vi "黑盾空调.vi"() -> ()   [LabVIEW 2016, in "环境动力监测库.lvlib" / "空调库.lvlib"]
uses:
  <vilib>/ptbypt/NI_PtbyPt.lvlib
panel:
  out "x+1":u32
  out "机柜空调告警状态":T1
  out "开关量输入状态解析":T2
  in  "解除告警":bool
  out "串口":string
  out "传感器状态":T3 {"系统模拟量量化数据"."电流" format="%#.2g"}
  in  "查看型号":bool
  in  "重开串口":bool
  in  "校时":bool
  in  "设定参数":bool
  in  "遥控":bool
  out "获取设备厂家信息":T4
  out "仪器时间":timestamp format="%<%Y/%m/%d %H:%M:%S>T"
  out "系统参数":T5
  out "写入缓冲区":string
  out "读取缓冲区":string
  out "读取选择":string(combo)
  out "通讯":bool=TRUE
  # "℃"
  # "℃"
  # "V"
  # "A"
  # "℃"
  # "℃"
  # "℃"
  # "℃"
  # "℃"
  # "℃"
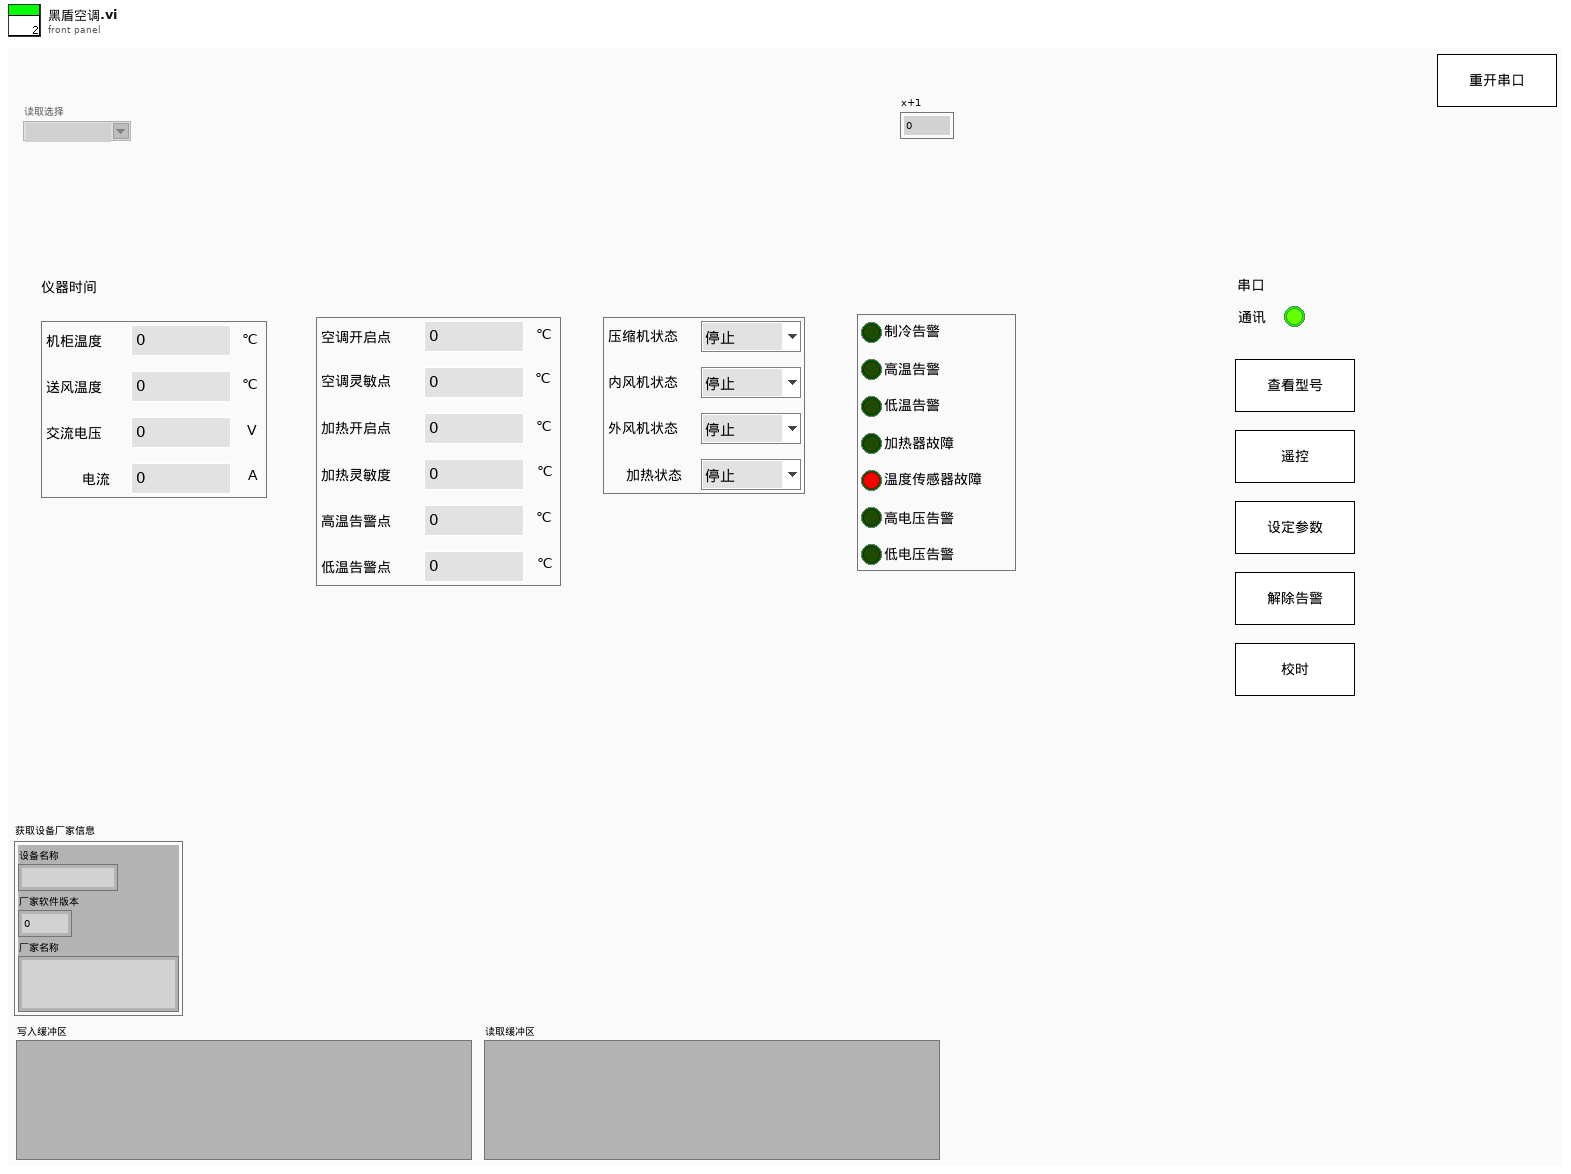
[diagram p1: front panel]
types:
  T1 = cluster{"制冷告警":bool, "高温告警":bool, "低温告警":bool, "加热器故障":bool, "温度传感器故障":bool, "高电压告警":bool, "低电压告警":bool, "预留":u16}
  T2 = cluster{"压缩机状态":enum16{"停止", "运行"}, "内风机状态":enum16{"停止", "运行"}, "外风机状态":enum16{"停止", "运行"}, "加热状态":enum16{"停止", "运行"}}
  T3 = cluster{"系统模拟量量化数据":cluster{"机柜温度":sgl, "送风温度":sgl, "交流电压":sgl, "电流":sgl}}
  T4 = cluster{"设备名称":string, "厂家软件版本":u16, "厂家名称":string}
  T5 = cluster{"空调开启点":u16, "空调灵敏点":u16, "加热开启点":u16, "加热灵敏度":u16, "高温告警点":u16, "低温告警点":u16}
  T6 = cluster{"分支":enum16{"open", "read", "write", "close"}, "字符串":string}
  T7 = cluster{"分支":enum16{"open", "read", "write", "close"}, "读取选择":string}
  T8 = cluster{"型号选择":enum16{"黑盾", "英维克", "仁科测控RS-KTC-N01"}, "MB session in":refnum<class "MB_Master.lvclass">, "英维克空调寄存器":u16[], "通讯状态":bool, "PORT":string, "IP":string, "Slave ID ":u8, "Serial Config":cluster{"baud rate (bps)":u32, "stop bits":u16, "parity":u16, "flow control":u16, "timeout":u32, "retries":i32}, "VISA Resource":refnum<visa-resource-name>, "MB通信方式选择":enum16{"串口", "TCP"}, "系统参数":cluster{"空调开启点":u16, "空调灵敏点":u16, "加热开启点":u16, "加热灵敏度":u16, "高温告警点":u16, "低温告警点":u16}}
  T9 = cluster{"温湿度":cluster{"状态":bool, "温度:":sgl, "湿度:":sgl, "详情  ":bool}, "空调":cluster{"状态":bool, "机柜温度:":sgl, "压缩机:":enum16{"停止", "运行"}, "电加热:":enum16{"停止", "运行"}, "详情  ":bool}, "排气扇":cluster{"排气扇":bool, "详情  ":bool}, "冰箱":cluster{"冰箱":bool, "详情  ":bool}}
  T10 = cluster{"漏水监测输出":cluster{"漏水监测告警":bool, "告警内容":string}, "门禁监测输出":cluster{"门禁监测告警":bool, "告警内容":string}, "门禁监测输出2":cluster{"门禁监测告警":bool, "告警内容":string}, "温湿度监测输出":cluster{"温湿度监测告警":bool, "告警内容":string}, "烟雾监测输出":cluster{"烟雾监测告警":bool, "告警内容":string}, "空调监测输出":cluster{"空调监测告警":bool, "告警内容":string}, "自动重合闸输出":cluster{"自动重合闸告警":bool, "告警内容":string}, "红外入侵输出":cluster{"红外入侵告警":bool, "告警内容":string}, "振动输出":cluster{"振动告警":bool, "告警内容":string}, "UPS输出":cluster{"UPS告警":bool, "告警内容":string}, "蓄电池输出":cluster{"蓄电池告警":bool, "告警内容":string}, "蓄电池输出2":cluster{"蓄电池告警":bool, "告警内容":string}, "GPS输出":cluster{"定位告警":bool, "告警内容":string}, "北斗输出":cluster{"定位告警":bool, "告警内容":string}, "气象输出":cluster{"气象告警":bool, "告警内容":string}, "废液输出":cluster{"废液告警":bool, "告警内容":string}, "废液输出2":cluster{"废液告警":bool, "告警内容":string}}
  T11 = enum32{"Bad", "Idle", "Run top level", "Running"}
  T12 = cluster{"机柜温度":sgl, "送风温度":sgl, "交流电压":sgl, "电流":sgl}
  T13 = cluster{"空调状态":enum16{"停止", "运行"}, "内风机状态":enum16{"停止", "运行"}, "外风机状态":enum16{"停止", "运行"}, "加热状态":enum16{"停止", "运行"}}
  T14 = enum16{"获取模拟量量化数据（浮点数）", "获取模拟量量化数据（定点数）", "获取开关输入状态", "获取机柜空调告警状态", "遥控", "获取系统参数（浮点数）", "获取系统参数（定点数）", "设定系统参数（浮点数）", "设定系统参数（定点数）", "获取系统历史数据（浮点数）", "获取系统历史数据（定点数）", "获取历史告警", "获取监测模块时间", "设定监测模块时间", "获取通信协议版本号", "获取设备地址", "获取设备厂家信息", "设定设备地址（ADR）"}
  T15 = enum16{"空调开机", "空调关机", "制冷开启", "制冷关闭", "制热开启", "制热关闭"}
  T16 = cluster{"分支":enum16{"open", "read", "write", "close"}, "连接的字符串":string}
  T17 = enum16{"空调开启点", "空调灵敏点", "加热开启点", "加热灵敏度", "高温告警点", "低温告警点"}
  T18 = enum16{"空调开启点", "空调灵敏点", "加热开启点", "加热灵敏度", "高温告警点", "低温告警点"}[]
  T19 = typedef "工况数据.ctl" = cluster{"time":string, "data":cluster{"ups":cluster{"ups":cluster{"input_voltage":ext, "input_frequency":ext, "output_voltage":ext, "output_current":ext, "output_frequency":ext, "output_active_power":ext, "output_apparent_power":ext, "load_rate":ext, "cabinet_temperature":ext, "battery_voltage":ext, "remaining_battery_capacity":ext, "power_on_status":string, "power_supply_mode":string, "fault":bool, "battery_low_voltage":bool, "mains_supply_abnormality":bool}, "启用":bool}, "air_conditioner":cluster{"air_conditioner":cluster{"cabinet_temperature":ext, "air_supply_temperature":ext, "voltage":ext, "current":ext, "compressor_status":string, "Internal_fan_status":string, "external_fan_status":string, "heating_state":string, "refrigeration_state":bool, "high_temperature_alarm":bool, "low_temperature_alarm":bool, "heater_fault":bool, "temperature_sensor_fault":bool, "high_voltage_alarm":bool, "low_voltage_alarm":bool, "refrigeration_start_point":ext, "refrigeration_sensitive_point":ext, "heating_start_point":ext, "heating_sensitive_point":ext, "high_temperature_alarm_point":ext, "low_temperature_alarm_point":ext}, "启用":bool}, "smoke_sensor":cluster{"smoke_sensor":cluster{"trigger_alarm":bool}, "启用":bool}, "water_immersion_sensor":cluster{"water_immersion_sensor":cluster{"trigger_alarm":bool}, "启用":bool}, "temperature_and_humidity_sensor":cluster{"temperature_and_humidity_sensor":cluster{"current_temperature":ext, "current_humidity":ext, "room_temperature_alarm":bool, "humidity_alarm":bool}, "启用":bool}, "gps":cluster{"gps":cluster{"current_longitude":ext, "current_latitude":ext, "launch_longitude":ext, "launch_latitude":ext, "shift_alarm":bool}, "启用":bool}, "solar_controller":cluster{"solar_controller":cluster{"array_voltage":ext, "array_current":ext, "generating_power":ext, "battery_voltage":dbl, "battery_current":ext, "ceiling_voltage":ext, "minimum_voltage":ext, "battery_temperature":ext, "remaining_battery_capacity":ext, "load_voltage":ext, "load_current":ext, "load_power":ext, "equipment_temperature":ext, "accumulated_electricity_consumption_of_the_day":ext, "accumulated_electricity_consumption_of_the_current_month":ext, "accumulated_electricity_consumption_in_the_current_year":ext, "total_accumulated_power_consumption":ext, "accumulated_charging_capacity_of_the_day":ext, "accumulated_charging_amount_of_the_current_month":ext, "accumulated_charging_capacity_of_the_current_year":ext, "total_cumulative_charge":ext}, "启用":bool}, "solar_controller_2":cluster{"solar_controller_2":cluster{"array_voltage":ext, "array_current":ext, "generating_power":ext, "battery_voltage":dbl, "battery_current":ext, "ceiling_voltage":ext, "minimum_voltage":ext, "battery_temperature":ext, "remaining_battery_capacity":ext, "load_voltage":ext, "load_current":ext, "load_power":ext, "equipment_temperature":ext, "accumulated_electricity_consumption_of_the_day":ext, "accumulated_electricity_consumption_of_the_current_month":ext, "accumulated_electricity_consumption_in_the_current_year":ext, "total_accumulated_power_consumption":ext, "accumulated_charging_capacity_of_the_day":ext, "accumulated_charging_amount_of_the_current_month":ext, "accumulated_charging_capacity_of_the_current_year":ext, "total_cumulative_charge":ext}, "启用":bool}, "NH3":cluster{"NH3":cluster{"F0":ext, "F1":ext, "syringe_temperature":ext, "alarm_step":dbl, "X0":ext}, "启用":bool}, "TP":cluster{"TP":cluster{"F0":ext, "F1":ext, "F2":ext, "F3":ext, "digestion_temperature":ext, "constant_temperature":ext, "syringe_temperature":ext, "alarm_step":dbl, "X0":ext}, "启用":bool}, "TN":cluster{"TN":cluster{"F0":ext, "F1":ext, "F2":ext, "F3":ext, "F4":ext, "F5":ext, "F6":ext, "F7":ext, "digestion_temperature":ext, "constant_temperature":ext, "syringe_temperature":ext, "alarm_step":dbl, "X0":ext}, "启用":bool}, "CODMn":cluster{"CODMn":cluster{"temperature_curve":ext[], "titration_curve":ext[], "F0":ext, "F1":ext, "F2":ext, "F3":ext, "F4":ext, "F5":ext, "A":ext, "B":ext, "K":ext}, "启用":bool}, "CODCr":cluster{"CODCr":cluster{"temperature_curve":ext[], "F0":ext, "F1":ext, "reagent_sensor":ext}, "启用":bool}}}
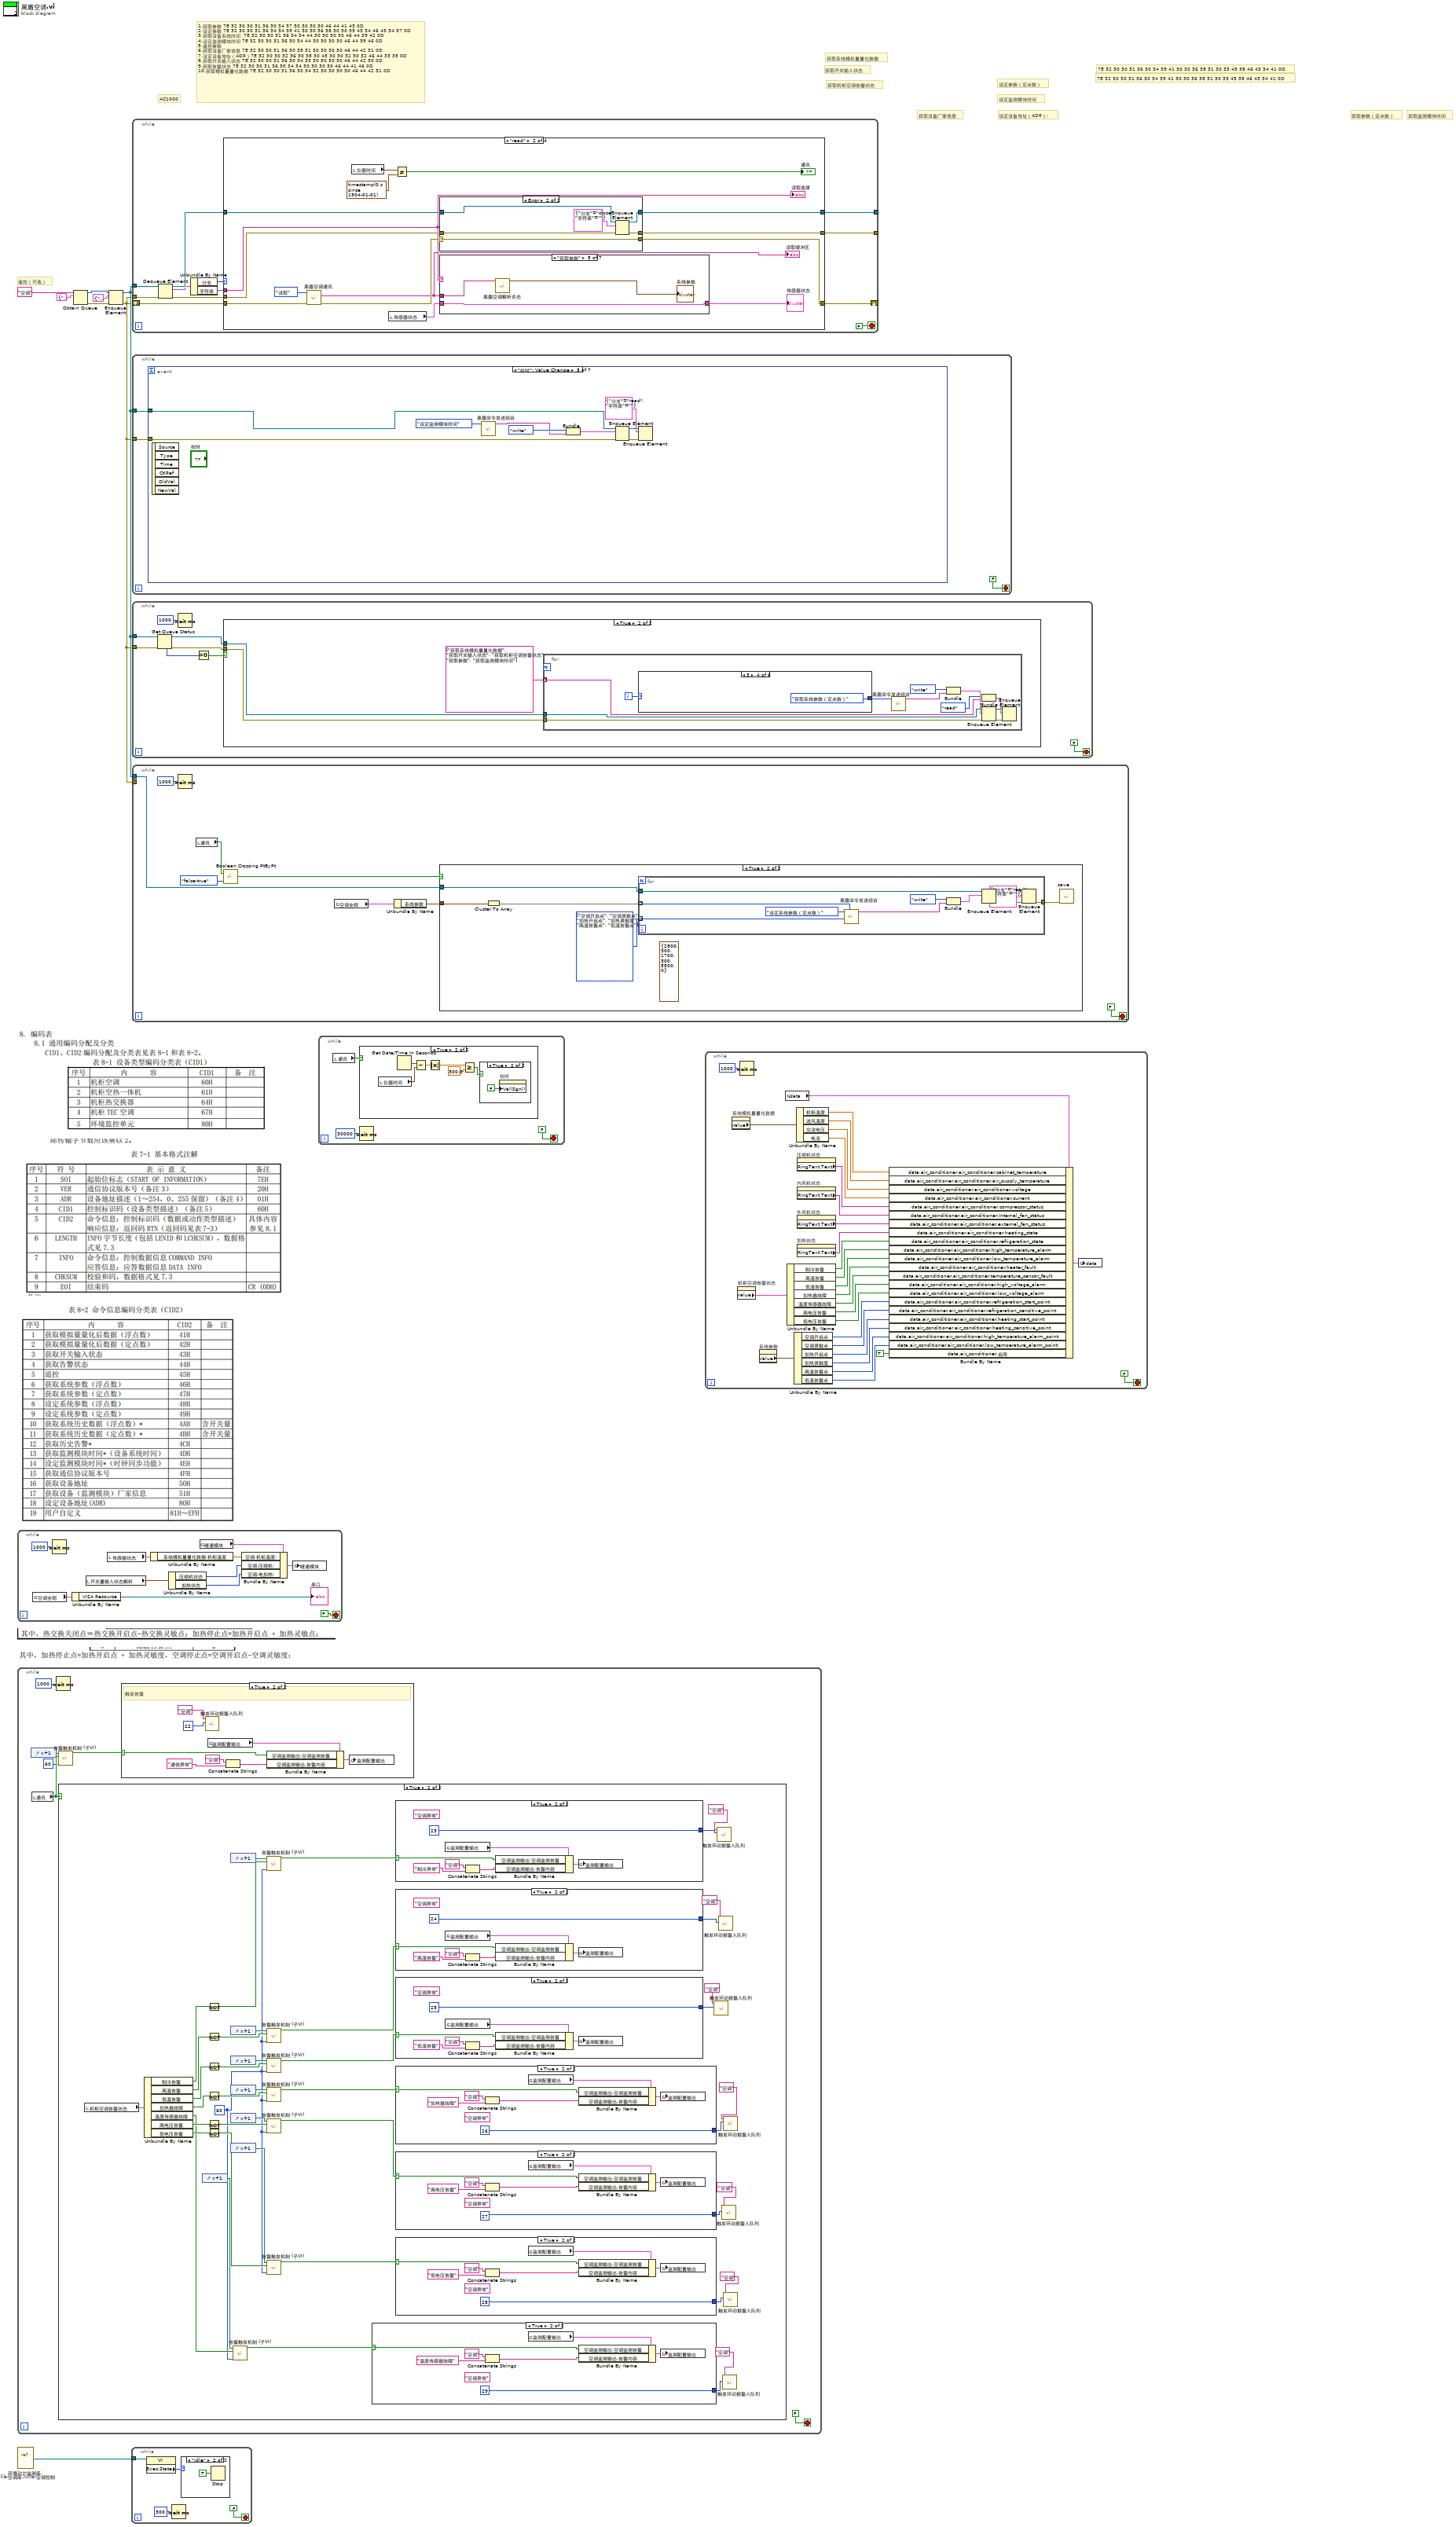
[diagram p0: block diagram]
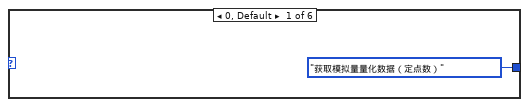
[diagram p16: hidden frame]
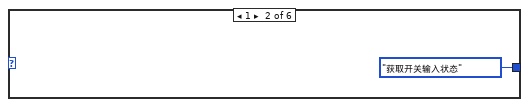
[diagram p17: hidden frame]
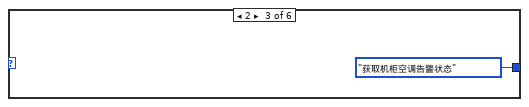
[diagram p18: hidden frame]
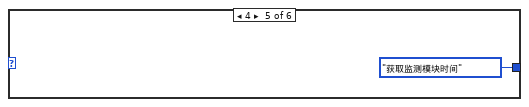
[diagram p19: hidden frame]
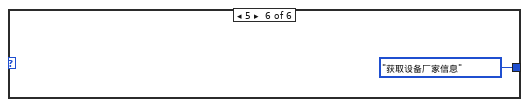
[diagram p20: hidden frame]
diagram:
  # "获取系统模拟量量化数据"
  # "设定设备地址（ADR）:"
  # "获取设备厂家信息"
  # "设定监测模块时间"
  # "获取监测模块时间"
  # "设定参数（定点数）"
  # "获取参数（定点数）"
  # "遥控（可选）"
  # "获取机柜空调告警状态"
  # "获取开关输入状态"
  # "7E 32 30 30 31 36 30 34 39 41 30 30 36 38 31 30 33 45 38 46 43 34 41 0D"
  # "7E 32 30 30 31 36 30 34 39 41 30 30 36 38 31 30 33 45 38 46 43 34 41 0D"
  # "AC1000"
  # "1.获取参数 7E 32 30 30 31 36 30 34 37 30 30 30 30 46 44 41 43 0D\n2.设定参数 7E 32 30 30 31 36 34 34 39 41 30 30 36 38 30 30 39 43 34 46 43 34 37 0D \n3.获取设备系统时间  7E 32 30 30 31 36 34 34 44 30 30 30 30 46 44 39 42 0D\n4.设定监测模块时间 7E 32 30 30 31 36 30 34 44 30 30 30 30 46 44 39 46 0D\n5.遥控参数\n6.获取设备厂家信息 7E 32 30 30 31 36 30 35 31 30 30 30 30 46 44 42 31 0D\n7.设定设备地址（ADR）7E 32 30 30 32 36 30 38 30 45 30 30 32 30 32 46 44 33 35 0D\n8.获取开关输入状态 7E 32 30 30 31 36 30 34 33 30 30 30 30 46 44 42 30 0D\n9.获取告警状态 7E 32 30 30 31 36 30 34 34 30 30 30 30 46 44 41 46 0D\n10.获取模拟量量化数据 7E 32 30 30 31 36 30 34 32 30 30 30 30 46 44 42 31 0D"
  n1 = while {
    stop <- FALSE stop-if-true
    n2 = global read "断电保存全局变量.vi" "空调全局"() -> (w10:T8)
    n3 = Wait (ms)(milliseconds to wait=u32 1000 ("等待时间（毫秒）")) -> ()  [unwired: 1 out]
    n4 = Unbundle By Name(w10) -> ("VISA Resource"=→"串口":refnum<visa-resource-name>)
    n5 = local read "开关量输入状态解析"() -> (w15:T2)
    n6 = local read "传感器状态"() -> (w13:T3)
    n7 = Unbundle By Name(w13) -> ("系统模拟量量化数据.机柜温度"=w14:sgl)
    n8 = Unbundle By Name(w15) -> ("压缩机状态"=w16:enum16{"停止", "运行"}, "加热状态"=w17:enum16{"停止", "运行"})
    n9 = global read "内部交互全局变量.vi" "暖通模块"() -> (w11:T9)
    n10 = Bundle By Name(cluster=w11, "空调.机柜温度:"=w14, "空调.压缩机:"=w16, "空调.电加热:"=w17) -> (w12:T9)
    n11 = global write "内部交互全局变量.vi" "暖通模块"(w12) -> ()
  }
  n12 = while {
    stop <- FALSE stop-if-true
    n13 = control-ref of="x+1"() -> (w21:refnum<vi>)
    n14 = local read "通讯"() -> (w22:bool)
    n15 = Wait (ms)(milliseconds to wait=u32 1000 ("等待时间（毫秒）")) -> ()  [unwired: 1 out]
    n16 = call "告警触发机制 (子VI).vi"("信号持续时间"=u32 60, "状态输出真-正常"=w22, "Digital输入"=w21) -> ("触发告警"=w23:bool)  [unwired: 6 in, 2 out]
    n17 = case shown="True" w22 {
      frame False {
      }
      frame True {
        w40 = u32 60 ("信号持续时间")
        n18 = local read "机柜空调告警状态"() -> (w68:T1)
        n19 = Unbundle By Name(w68) -> ("制冷告警"=w64:bool, "高温告警"=w58:bool, "低温告警"=w55:bool, "加热器故障"=w51:bool, "温度传感器故障"=w42:bool, "高电压告警"=w47:bool, "低电压告警"=w45:bool)
        n20 = control-ref of="x+1"() -> (w43:refnum<vi>)
        n21 = Not(x=w64) -> (.not. x?=w65:bool)
        n22 = Not(x=w58) -> (.not. x?=w61:bool)
        n23 = Not(x=w55) -> (.not. x?=w57:bool)
        n24 = Not(x=w51) -> (.not. x?=w53:bool)
        n25 = Not(x=w47) -> (.not. x?=w49:bool)
        n26 = Not(x=w45) -> (.not. x?=w62:bool)
        n27 = control-ref of="x+1"() -> (w66:refnum<vi>)
        n28 = control-ref of="x+1"() -> (w60:refnum<vi>)
        n29 = control-ref of="x+1"() -> (w56:refnum<vi>)
        n30 = control-ref of="x+1"() -> (w52:refnum<vi>)
        n31 = control-ref of="x+1"() -> (w48:refnum<vi>)
        n32 = control-ref of="x+1"() -> (w67:refnum<vi>)
        n33 = call "告警触发机制 (子VI).vi"("信号持续时间"=w40, "状态输出真-正常"=w42, "Digital输入"=w43) -> ("触发告警"=w41:bool)  [unwired: 6 in, 2 out]
        n34 = call "告警触发机制 (子VI).vi"("信号持续时间"=w40, "状态输出真-正常"=w65, "Digital输入"=w66) -> ("触发告警"=w63:bool)  [unwired: 6 in, 2 out]
        n35 = call "告警触发机制 (子VI).vi"("信号持续时间"=w40, "状态输出真-正常"=w61, "Digital输入"=w60) -> ("触发告警"=w59:bool)  [unwired: 6 in, 2 out]
        n36 = call "告警触发机制 (子VI).vi"("信号持续时间"=w40, "状态输出真-正常"=w57, "Digital输入"=w56) -> ("触发告警"=w54:bool)  [unwired: 6 in, 2 out]
        n37 = call "告警触发机制 (子VI).vi"("信号持续时间"=w40, "状态输出真-正常"=w53, "Digital输入"=w52) -> ("触发告警"=w50:bool)  [unwired: 6 in, 2 out]
        n38 = call "告警触发机制 (子VI).vi"("信号持续时间"=w40, "状态输出真-正常"=w49, "Digital输入"=w48) -> ("触发告警"=w46:bool)  [unwired: 6 in, 2 out]
        n39 = call "告警触发机制 (子VI).vi"("信号持续时间"=w40, "状态输出真-正常"=w62, "Digital输入"=w67) -> ("触发告警"=w44:bool)  [unwired: 6 in, 2 out]
        n40 = case shown="True" w41 {
          selector: w41 -> [_ w86]
          tunnel: [_ 29 ("code")] -> w26
          frame False {
          }
          frame True {
            (unwired) "空调异常" ("设备")
            n41 = Concatenate Strings("空调" ("设备"), "温度传感器故障" ("日志信息")) -> (w85:string)
            n42 = global read "内部交互全局变量.vi" "监测配置输出"() -> (w88:T10)
            n43 = Bundle By Name(cluster=w88, "空调监测输出.空调监测告警"=w86, "空调监测输出.告警内容"=w85) -> (w87:T10)
            n44 = global write "内部交互全局变量.vi" "监测配置输出"(w87) -> ()
          }
        }
        n45 = case shown="True" w63 {
          selector: w63 -> [_ w114]
          tunnel: [_ 23 ("code")] -> w39
          frame False {
          }
          frame True {
            (unwired) "空调异常" ("设备")
            n46 = global read "内部交互全局变量.vi" "监测配置输出"() -> (w116:T10)
            n47 = Concatenate Strings("空调" ("设备"), "制冷异常" ("日志信息")) -> (w113:string)
            n48 = Bundle By Name(cluster=w116, "空调监测输出.空调监测告警"=w114, "空调监测输出.告警内容"=w113) -> (w115:T10)
            n49 = global write "内部交互全局变量.vi" "监测配置输出"(w115) -> ()
          }
        }
        n50 = case shown="True" w59 {
          selector: w59 -> [_ w107]
          tunnel: [_ 24 ("code")] -> w36
          frame False {
          }
          frame True {
            (unwired) "空调异常" ("设备")
            n51 = global read "内部交互全局变量.vi" "监测配置输出"() -> (w109:T10)
            n52 = Concatenate Strings("空调" ("设备"), "高温告警" ("日志信息")) -> (w106:string)
            n53 = Bundle By Name(cluster=w109, "空调监测输出.空调监测告警"=w107, "空调监测输出.告警内容"=w106) -> (w108:T10)
            n54 = global write "内部交互全局变量.vi" "监测配置输出"(w108) -> ()
          }
        }
        n55 = case shown="True" w54 {
          selector: w54 -> [_ w100]
          tunnel: [_ 25 ("code")] -> w35
          frame False {
          }
          frame True {
            (unwired) "空调异常" ("设备")
            n56 = global read "内部交互全局变量.vi" "监测配置输出"() -> (w102:T10)
            n57 = Concatenate Strings("空调" ("设备"), "低温告警" ("日志信息")) -> (w99:string)
            n58 = Bundle By Name(cluster=w102, "空调监测输出.空调监测告警"=w100, "空调监测输出.告警内容"=w99) -> (w101:T10)
            n59 = global write "内部交互全局变量.vi" "监测配置输出"(w101) -> ()
          }
        }
        n60 = case shown="True" w50 {
          selector: w50 -> [_ w93]
          tunnel: [_ 26 ("code")] -> w32
          frame False {
          }
          frame True {
            (unwired) "空调异常" ("设备")
            n61 = Concatenate Strings("空调" ("设备"), "加热器故障" ("日志信息")) -> (w92:string)
            n62 = global read "内部交互全局变量.vi" "监测配置输出"() -> (w95:T10)
            n63 = Bundle By Name(cluster=w95, "空调监测输出.空调监测告警"=w93, "空调监测输出.告警内容"=w92) -> (w94:T10)
            n64 = global write "内部交互全局变量.vi" "监测配置输出"(w94) -> ()
          }
        }
        n65 = case shown="True" w46 {
          selector: w46 -> [_ w79]
          tunnel: [_ 27 ("code")] -> w31
          frame False {
          }
          frame True {
            (unwired) "空调异常" ("设备")
            n66 = Concatenate Strings("空调" ("设备"), "高电压告警" ("日志信息")) -> (w78:string)
            n67 = global read "内部交互全局变量.vi" "监测配置输出"() -> (w81:T10)
            n68 = Bundle By Name(cluster=w81, "空调监测输出.空调监测告警"=w79, "空调监测输出.告警内容"=w78) -> (w80:T10)
            n69 = global write "内部交互全局变量.vi" "监测配置输出"(w80) -> ()
          }
        }
        n70 = case shown="True" w44 {
          selector: w44 -> [_ w71]
          tunnel: [_ 28 ("code")] -> w28
          frame False {
          }
          frame True {
            (unwired) "空调异常" ("设备")
            n71 = Concatenate Strings("空调" ("设备"), "低电压告警" ("日志信息")) -> (w72:string)
            n72 = global read "内部交互全局变量.vi" "监测配置输出"() -> (w74:T10)
            n73 = Bundle By Name(cluster=w74, "空调监测输出.空调监测告警"=w71, "空调监测输出.告警内容"=w72) -> (w73:T10)
            n74 = global write "内部交互全局变量.vi" "监测配置输出"(w73) -> ()
          }
        }
        n75 = call "触发环动报警入队列.vi"("code"=w35, "元器件"="空调") -> ()  [unwired: 10 in]
        n76 = call "触发环动报警入队列.vi"("code"=w39, "元器件"="空调") -> ()  [unwired: 10 in]
        n77 = call "触发环动报警入队列.vi"("code"=w36, "元器件"="空调") -> ()  [unwired: 10 in]
        n78 = call "触发环动报警入队列.vi"("code"=w31, "元器件"="空调") -> ()  [unwired: 10 in]
        n79 = call "触发环动报警入队列.vi"("code"=w26, "元器件"="空调") -> ()  [unwired: 10 in]
        n80 = call "触发环动报警入队列.vi"("code"=w32, "元器件"="空调") -> ()  [unwired: 10 in]
        n81 = call "触发环动报警入队列.vi"("code"=w28, "元器件"="空调") -> ()  [unwired: 10 in]
      }
    }
    n82 = case shown="True" w23 {
      selector: w23 -> [_ w125]
      frame False {
      }
      frame True {
        # "触发告警"
        n83 = call "触发环动报警入队列.vi"("code"=22, "元器件"="空调" ("设备")) -> ()  [unwired: 10 in]
        n84 = global read "内部交互全局变量.vi" "监测配置输出"() -> (w124:T10)
        n85 = Concatenate Strings("空调" ("设备"), "通信异常" ("设备")) -> (w121:string)
        n86 = Bundle By Name(cluster=w124, "空调监测输出.空调监测告警"=w125, "空调监测输出.告警内容"=w121) -> (w123:T10)
        n87 = global write "内部交互全局变量.vi" "监测配置输出"(w123) -> ()
      }
    }
  }
  n88 = vi-ref "环境动力监测库.lvlib:空调库.lvlib:空调控制.vi"() -> (w3:refnum<vi>)
  n89 = Obtain Queue(name (unnamed)="空调" ("名称（未命名）"), element data type=T6 {"分支"=enum."open", "字符串"="获取系统模拟量量化数据"}) -> (queue out=w7:refnum<queue>, error out=w6:errorcluster)  [unwired: 3 in, 1 out]
  n90 = Enqueue Element(queue=w7, element=T7 {"分支"=enum."open", "读取选择"="获取系统模拟量量化数据"}, error in (no error)=w6) -> (queue out=w2:refnum<queue>, error out=w1:errorcluster)  [unwired: 1 in, 1 out]
  n91 = while {
    tunnel: w3 -> [w129]
    stop <- FALSE stop-if-true
    n92 = property class="VI"(reference=w129) -> ("Exec.State"=w128:T11)  [unwired: 1 in, 2 out]
    n93 = Wait (ms)(milliseconds to wait=u32 300 ("等待时间（毫秒）")) -> ()  [unwired: 1 out]
    n94 = case shown="\"Idle\"" w128 {
      frame "Bad", Default {
      }
      frame "Idle" {
        n95 = Stop(stop? (T)=TRUE ("停止？(T)")) -> ()
      }
    }
  }
  n96 = while {
    tunnel: w2 -> [w141]
    tunnel: w1 -> [w140]
    shift-right: [w139] -> _
    shift-left: w1 -> [w138]
    tunnel: [w135] -> _
    tunnel: [w134] -> _
    stop <- FALSE stop-if-true
    n97 = Dequeue Element(queue=w141, error in (no error)=w140) -> (queue out=w137:refnum<queue>, element=w133:T6, error out=w136:errorcluster)  [unwired: 1 in, 1 out]
    n98 = Unbundle By Name(w133) -> ("分支"=w132:enum16{"open", "read", "write", "close"}, "字符串"=w131:string)
    n99 = case shown="\"read\"" w132 {
      tunnel: [w147 w154 w196 w204] -> w139
      tunnel: w138 -> [_ w162 w197 w205]
      tunnel: w137 -> [w146 w158 w194 w203]
      tunnel: w136 -> [w145 w156 w193 w202]
      tunnel: [w146 w157 w194 w200] -> w135
      tunnel: [w145 w155 w193 w199] -> w134
      tunnel: w131 -> [_ w161 w195 _]
      frame "open", Default {
        n100 = global read "断电保存全局变量.vi" "空调全局"() -> (w144:T8)
        n101 = Unbundle By Name(w144) -> ("VISA Resource"=w143:refnum<visa-resource-name>)
        n102 = call "黑盾空调通讯.vi"("VISA resource name"=w143, "功能输入"=enum16{"打开串口", "写入", "读取", "关闭串口"}."打开串口") -> ("error out"=w147:errorcluster)  [unwired: 7 in, 2 out]
      }
      frame "read" {
        n103 = call "黑盾空调通讯.vi"("error in (no error)"=w162, "功能输入"=enum16{"打开串口", "写入", "读取", "关闭串口"}."读取") -> ("error out"=w159:errorcluster, "读取缓冲区"=w153:string)  [unwired: 7 in, 1 out]
        "读取缓冲区" <- w153
        n104 = local read "仪器时间"() -> (w149:timestamp)
        n105 = local read "传感器状态"() -> (w160:T3)
        n106 = Not Equal?(x=w149, y=timestamp(0 s since 1904-01-01)) -> (x != y?=→"通讯":bool)
        n107 = case shown="Error" w159 {
          selector: w159 -> [w166 w167]
          tunnel: w158 -> [w165 w171]
          tunnel: [w165 w170] -> w157
          tunnel: w156 -> [w164 w169]
          tunnel: [w164 w168] -> w155
          tunnel: [w166 w167] -> w154
          frame No Error {
          }
          frame Error {
            n108 = Enqueue Element(queue=w171, element=T6 {"分支"=enum."close", "字符串"=""} ("元素"), error in (no error)=w169) -> (queue out=w170:refnum<queue>, error out=w168:errorcluster)  [unwired: 1 in, 1 out]
          }
        }
        n109 = case shown="\"获取参数\"" w161 {
          tunnel: w153 -> [_ w177 w180 w183 w186 w189 w192]
          tunnel: w160 -> [w173 w176 w178 w182 w184 w188 w190]
          tunnel: [w173 w174 w178 w182 w184 w188 w190] -> w152
          frame "假", Default {
          }
          frame "获取系统模拟量量化数据" {
            n110 = call-poly "黑盾空调解析多态.vi"("输入字符串"=w177) -> ("系统模拟量量化数据"=w175:T12)  [unwired: 10 in]
            n111 = Bundle By Name(cluster=w176, "系统模拟量量化数据"=w175) -> (w174:T3)
          }
          frame "获取开关输入状态" {
            n112 = call-poly "黑盾空调解析多态.vi"("输入字符串"=w180) -> ("开关量输入状态解析"=→"开关量输入状态解析":T13)  [unwired: 10 in]
          }
          frame "获取机柜空调告警状态" {
            n113 = call-poly "黑盾空调解析多态.vi"("输入字符串"=w183) -> ("机柜空调告警状态"=→"机柜空调告警状态":T1)  [unwired: 10 in]
          }
          frame "获取参数" {
            n114 = call-poly "黑盾空调解析多态.vi"("输入字符串"=w186) -> ("获取参数(定点数)"=→"系统参数":T5)  [unwired: 10 in]
          }
          frame "获取监测模块时间" {
            n115 = call-poly "黑盾空调解析多态.vi"("输入字符串"=w189) -> ("时间标识"=→"仪器时间":timestamp)  [unwired: 10 in]
          }
          frame "获取设备厂家信息" {
            n116 = call-poly "黑盾空调解析多态.vi"("输入字符串"=w192) -> ("获取设备厂家信息"=→"获取设备厂家信息":T4)  [unwired: 10 in]
          }
        }
        "传感器状态" <- w152
        "读取选择" <- w161
      }
      frame "write" {
        n117 = call "黑盾空调通讯.vi"("error in (no error)"=w197, "写入缓冲区"=w195, "功能输入"=enum16{"打开串口", "写入", "读取", "关闭串口"}."写入") -> ("error out"=w196:errorcluster)  [unwired: 6 in, 2 out]
        "写入缓冲区" <- w195
      }
      frame "close" {
        n118 = call "黑盾空调通讯.vi"("error in (no error)"=w205, "功能输入"=enum16{"打开串口", "写入", "读取", "关闭串口"}."关闭串口") -> ("error out"=w204:errorcluster)  [unwired: 7 in, 2 out]
        n119 = Enqueue Element(queue=w203, element=T6 {"分支"=enum."open", "字符串"=""} ("元素"), error in (no error)=w202) -> (queue out=w200:refnum<queue>, error out=w199:errorcluster)  [unwired: 1 in, 1 out]
      }
    }
  }
  n120 = while {
    tunnel: w2 -> [w208]
    tunnel: w1 -> [w207]
    stop <- FALSE stop-if-true
    n121 = event shown="[4] \"校时\": Value Change" {
      selector: _ -> [_ _ _ _ _ _ _]
      dyn-events: _ -> [_ _ _ _ _ _ _]
      timeout: _ -> [_ _ _ _ _ _ _]
      tunnel: w208 -> [_ w215 w234 w253 w288 _ _]
      tunnel: w207 -> [_ w214 w235 w252 w287 _ _]
      event Timeout {
        n122 = event-data() -> ()  [unwired: 1 in, 3 out]
      }
      event "重开串口": Value Change {
        n123 = event-data() -> ()  [unwired: 1 in, 6 out]
        n124 = global read "断电保存全局变量.vi" "空调全局"() -> (w210:T8)
        n125 = Unbundle By Name(w210) -> ("VISA Resource"=w213:refnum<visa-resource-name>, "IP"=w212:string, "PORT"=w211:string)
        n126 = call "串口配置.vi"("PORT"=w211, "IP"=w212, "请选择串口:"=w213) -> ("PORT 2"=w216:string, "IP 2"=w217:string, "确认 2"=w218:bool, "VISA资源名称 2"=w219:refnum<visa-resource-name>)  [unwired: 5 in]
        n127 = case shown="True" w218 {
          tunnel: w219 -> [_ w223]
          tunnel: w215 -> [_ w225]
          tunnel: w214 -> [_ w224]
          tunnel: w217 -> [_ w222]
          tunnel: w216 -> [_ w221]
          tunnel: w210 -> [_ w220]
          frame False {
          }
          frame True {
            n128 = flat-sequence {
              tunnel: w225 -> [w233]
              tunnel: w224 -> [w232]
              tunnel: w223 -> [w229]
              tunnel: w222 -> [w228]
              tunnel: w221 -> [w227]
              tunnel: w220 -> [w230]
              frame #0 {
                n129 = Bundle By Name(cluster=w230, "VISA Resource"=w229, "IP"=w228, "PORT"=w227) -> (w226:T8)
                n130 = global write "断电保存全局变量.vi" "空调全局"(w226) -> ()
                n131 = Enqueue Element(queue=w233, element=T6 {"分支"=enum."close", "字符串"=""} ("元素"), error in (no error)=w232) -> ()  [unwired: 1 in, 3 out]
              }
              frame #1 {
                n132 = call "save.vi"() -> ()  [unwired: 11 in, 1 out]
              }
            }
          }
        }
      }
      event "遥控": Value Change {
        n133 = event-data() -> ()  [unwired: 1 in, 6 out]
        n134 = call "遥控参数对话框.vi"() -> ("遥控参数选择输出"=w236:T15, "确定?"=w237:bool)  [unwired: 10 in]
        n135 = case shown="True" w237 {
          tunnel: w236 -> [_ w246]
          tunnel: w235 -> [_ w245]
          tunnel: w234 -> [_ w244]
          frame False {
          }
          frame True {
            n136 = call "黑盾命令发送组合.vi"("遥控参数选择"=w246, "CID2枚举"=T14."遥控") -> ("连接的字符串"=w242:string)  [unwired: 9 in]
            n137 = Bundle("分支"=enum16{"open", "read", "write", "close"}."write", "连接的字符串"=w242) -> (w241:T16)  [unwired: 1 in]
            n138 = Enqueue Element(queue=w244, element=w241, error in (no error)=w245) -> (queue out=w240:refnum<queue>, error out=w239:errorcluster)  [unwired: 1 in, 1 out]
            n139 = Enqueue Element(queue=w240, element=T6 {"分支"=enum."read", "字符串"=""} ("元素"), error in (no error)=w239) -> ()  [unwired: 1 in, 3 out]
          }
        }
      }
      event "设定参数": Value Change {
        n140 = event-data() -> ()  [unwired: 1 in, 6 out]
        n141 = local read "系统参数"() -> (w248:T5)
        n142 = call "设定参数对话框.vi"("获取参数(定点数)"=w248) -> ("参数 2"=w249:u16, "设定参数（定点数）选择 2"=w250:T17, "确定?"=w251:bool)  [unwired: 8 in]
        n143 = case shown="True" w251 {
          tunnel: w252 -> [_ w263]
          tunnel: w253 -> [_ w262]
          tunnel: w250 -> [_ w255]
          tunnel: w249 -> [_ w254]
          frame False {
          }
          frame True {
            n144 = flat-sequence {
              tunnel: w255 -> [w268]
              tunnel: w254 -> [w265]
              frame #0 {
                n145 = global read "断电保存全局变量.vi" "空调全局"() -> (w267:T8)
                n146 = case shown="\"低温告警点\"" w268 {
                  tunnel: w267 -> [w271 w273 w276 w279 w282 w285]
                  tunnel: w265 -> [w270 w274 w277 w280 w283 w286]
                  tunnel: [w269 w272 w275 w278 w281 w284] -> w266
                  frame "空调开启点", Default {
                    n147 = Bundle By Name(cluster=w271, "系统参数.空调开启点"=w270) -> (w269:T8)
                  }
                  frame "空调灵敏点" {
                    n148 = Bundle By Name(cluster=w273, "系统参数.空调灵敏点"=w274) -> (w272:T8)
                  }
                  frame "加热开启点" {
                    n149 = Bundle By Name(cluster=w276, "系统参数.加热开启点"=w277) -> (w275:T8)
                  }
                  frame "加热灵敏度" {
                    n150 = Bundle By Name(cluster=w279, "系统参数.加热灵敏度"=w280) -> (w278:T8)
                  }
                  frame "高温告警点" {
                    n151 = Bundle By Name(cluster=w282, "系统参数.高温告警点"=w283) -> (w281:T8)
                  }
                  frame "低温告警点" {
                    n152 = Bundle By Name(cluster=w285, "系统参数.低温告警点"=w286) -> (w284:T8)
                  }
                }
                n153 = global write "断电保存全局变量.vi" "空调全局"(w266) -> ()
              }
              frame #1 {
                n154 = call "save.vi"() -> ()  [unwired: 11 in, 1 out]
              }
            }
            n155 = call "黑盾命令发送组合.vi"("参数"=w254, "设定参数（定点数）选择"=w255, "CID2枚举"=T14."设定系统参数（定点数）") -> ("连接的字符串"=w260:string)  [unwired: 8 in]
            n156 = Bundle("分支"=enum16{"open", "read", "write", "close"}."write", "连接的字符串"=w260) -> (w259:T16)  [unwired: 1 in]
            n157 = Enqueue Element(queue=w262, element=w259, error in (no error)=w263) -> (queue out=w258:refnum<queue>, error out=w257:errorcluster)  [unwired: 1 in, 1 out]
            n158 = Enqueue Element(queue=w258, element=T6 {"分支"=enum."read", "字符串"=""} ("元素"), error in (no error)=w257) -> ()  [unwired: 1 in, 3 out]
          }
        }
      }
      event "校时": Value Change {
        n159 = event-data() -> ()  [unwired: 1 in, 6 out]
        n160 = call "黑盾命令发送组合.vi"("CID2枚举"=T14."设定监测模块时间") -> ("连接的字符串"=w293:string)  [unwired: 10 in]
        n161 = Bundle("分支"=enum16{"open", "read", "write", "close"}."write", "连接的字符串"=w293) -> (w292:T16)  [unwired: 1 in]
        n162 = Enqueue Element(queue=w288, element=w292, error in (no error)=w287) -> (queue out=w291:refnum<queue>, error out=w290:errorcluster)  [unwired: 1 in, 1 out]
        n163 = Enqueue Element(queue=w291, element=T6 {"分支"=enum."read", "字符串"=""} ("元素"), error in (no error)=w290) -> ()  [unwired: 1 in, 3 out]
      }
      event "查看型号": Value Change {
        n164 = event-data() -> ()  [unwired: 1 in, 6 out]
        n165 = One Button Dialog(message="空调品牌为:黑盾" ("消息")) -> ()  [unwired: 1 in, 1 out]
      }
      event "解除告警": Value Change {
        n166 = event-data() -> ()  [unwired: 1 in, 6 out]
        n167 = global read "内部交互全局变量.vi" "监测配置输出"() -> (w298:T10)
        n168 = Bundle By Name(cluster=w298, "空调监测输出.空调监测告警"=FALSE) -> (w297:T10)
        n169 = global write "内部交互全局变量.vi" "监测配置输出"(w297) -> ()
        "x+1" <- u32 0 ("x+1")
      }
    }
  }
  n170 = while {
    tunnel: w2 -> [w307]
    tunnel: w1 -> [w306]
    stop <- FALSE stop-if-true
    n171 = Get Queue Status(queue=w307, error in (no error)=w306) -> (queue out=w303:refnum<queue>, error out=w302:errorcluster, # elements in queue=w305:i32)  [unwired: 1 in, 5 out]
    n172 = Wait (ms)(milliseconds to wait=u32 1000 ("等待时间（毫秒）")) -> ()  [unwired: 1 out]
    n173 = Equal To 0?(x=w305) -> (x = 0?=w304:bool)
    n174 = case shown="True" w304 {
      tunnel: w303 -> [_ w310]
      tunnel: w302 -> [_ w309]
      frame False {
      }
      frame True {
        n175 = for {
          tunnel: string[] ["获取系统模拟量量化数据", "获取开关输入状态", "获取机柜空调告警状态", "获取参数", "获取监测模块时间"] -> [w313] mode=indexing
          tunnel: w310 -> [w323]
          tunnel: w309 -> [w322]
          i -> [w321]
          n176 = case shown="3" w321 {
            tunnel: [T14."获取模拟量量化数据（定点数）" ("CID2枚举") T14."获取开关输入状态" ("CID2枚举") T14."获取机柜空调告警状态" ("CID2枚举") T14."获取系统参数（定点数）" ("CID2枚举") T14."获取监测模块时间" ("CID2枚举") T14."获取设备厂家信息" ("CID2枚举")] -> w320
            frame 0, Default {
            }
            frame 1 {
            }
            frame 2 {
            }
            frame 3 {
            }
            frame 4 {
            }
            frame 5 {
            }
          }
          n177 = call "黑盾命令发送组合.vi"("CID2枚举"=w320) -> ("连接的字符串"=w318:string)  [unwired: 10 in]
          n178 = Bundle("分支"=enum16{"open", "read", "write", "close"}."write", "连接的字符串"=w318) -> (w317:T16)  [unwired: 1 in]
          n179 = Bundle("分支"=enum16{"open", "read", "write", "close"}."read", "读取选择"=w313) -> (w312:T7)  [unwired: 1 in]
          n180 = Enqueue Element(queue=w323, element=w317, error in (no error)=w322) -> (queue out=w315:refnum<queue>, error out=w314:errorcluster)  [unwired: 1 in, 1 out]
          n181 = Enqueue Element(queue=w315, element=w312, error in (no error)=w314) -> ()  [unwired: 1 in, 3 out]
        }
      }
    }
  }
  n182 = while {
    tunnel: w1 -> [_]
    tunnel: w2 -> [w333]
    stop <- FALSE stop-if-true
    n183 = Wait (ms)(milliseconds to wait=u32 1000 ("等待时间（毫秒）")) -> ()  [unwired: 1 out]
    n184 = local read "通讯"() -> (w335:bool)
    n185 = call <vilib>:"Boolean Crossing PtByPt.vi"("direction"=enum16{"either", "false-true", "true-false"}."false-true", "input"=w335) -> ("crossing"=w330:bool)  [unwired: 1 in]
    n186 = global read "断电保存全局变量.vi" "空调全局"() -> (w332:T8)
    n187 = Unbundle By Name(w332) -> ("系统参数"=w331:T5)
    n188 = case shown="True" w330 {
      tunnel: w333 -> [_ w340]
      tunnel: w331 -> [_ w338]
      frame False {
      }
      frame True {
        w341 = T18 [enum."空调开启点", enum."空调灵敏点", enum."加热开启点", enum."加热灵敏度", enum."高温告警点", enum."低温告警点"] items=["空调开启点", "空调灵敏点", "加热开启点", "加热灵敏度", "高温告警点", "低温告警点"]
        (unwired) T5 {"空调开启点"=2800, "空调灵敏点"=300, "加热开启点"=1700, "加热灵敏度"=300, "高温告警点"=5500, "低温告警点"=0} ("系统参数")
        n189 = Cluster To Array(cluster=w338) -> (array=w342:u16[])
        n190 = for {
          tunnel: w342 -> [w352] mode=indexing
          tunnel: w341 -> [w353] mode=indexing
          tunnel: w340 -> [w351]
          tunnel: [w343] -> w339
          n191 = call "黑盾命令发送组合.vi"("参数"=w352, "设定参数（定点数）选择"=w353, "CID2枚举"=T14."设定系统参数（定点数）") -> ("连接的字符串"=w349:string)  [unwired: 8 in]
          n192 = Bundle("分支"=enum16{"open", "read", "write", "close"}."write", "连接的字符串"=w349) -> (w350:T16)  [unwired: 1 in]
          n193 = Enqueue Element(queue=w351, element=w350) -> (queue out=w345:refnum<queue>, error out=w344:errorcluster)  [unwired: 2 in, 1 out]
          n194 = Enqueue Element(queue=w345, element=T6 {"分支"=enum."read", "字符串"=""} ("元素"), error in (no error)=w344) -> (error out=w343:errorcluster)  [unwired: 1 in, 2 out]
        }
        n195 = call "save.vi"("error in (no error)"=w339) -> ()  [unwired: 10 in, 1 out]
      }
    }
  }
  n196 = while {
    stop <- FALSE stop-if-true
    n197 = local read "通讯"() -> (w354:bool)
    n198 = case shown="True" w354 {
      frame False {
      }
      frame True {
        n199 = local read "仪器时间"() -> (w361:timestamp)
        n200 = Get Date/Time In Seconds() -> (seconds since 1Jan1904=w362:timestamp)
        n201 = Subtract(x=w362, y=w361) -> (x-y=w360:dbl)
        n202 = Absolute Value(x=w360) -> (abs(x)=w359:dbl)
        n203 = Greater Or Equal?(x=w359, y=300.0) -> (x >= y?=w357:bool)
        n204 = case shown="True" w357 {
          frame False {
          }
          frame True {
            n205 = property on="校时" class="Bool (strict)"("Val(Sgnl)"=FALSE) -> ()  [unwired: 2 in, 2 out]
          }
        }
      }
    }
    n206 = Wait (ms)(milliseconds to wait=u32 30000 ("等待时间（毫秒）")) -> ()  [unwired: 1 out]
  }
  n207 = while {
    stop <- FALSE stop-if-true
    n208 = property on="系统模拟量量化数据" class="Clust (strict)"() -> ("Value"=w388:T12)  [unwired: 2 in, 2 out]
    n209 = property on="机柜空调告警状态" class="Clust (strict)"() -> ("Value"=w379:T1)  [unwired: 2 in, 2 out]
    n210 = Wait (ms)(milliseconds to wait=u32 1000 ("等待时间（毫秒）")) -> ()  [unwired: 1 out]
    n211 = property on="系统参数" class="Clust (strict)"() -> ("Value"=w371:T5)  [unwired: 2 in, 2 out]
    n212 = global read "工况数据接口全局.vi" "data"() -> (w392:T19)
    n213 = Unbundle By Name(w379) -> ("制冷告警"=w378:bool, "高温告警"=w377:bool, "低温告警"=w376:bool, "加热器故障"=w375:bool, "温度传感器故障"=w374:bool, "高电压告警"=w373:bool, "低电压告警"=w372:bool)
    n214 = Unbundle By Name(w371) -> ("空调开启点"=w370:u16, "空调灵敏点"=w369:u16, "加热开启点"=w368:u16, "加热灵敏度"=w367:u16, "高温告警点"=w366:u16, "低温告警点"=w365:u16)
    n215 = Unbundle By Name(w388) -> ("机柜温度"=w387:sgl, "送风温度"=w386:sgl, "交流电压"=w385:sgl, "电流"=w384:sgl)
    n216 = property on="压缩机状态" class="Enum (strict)"() -> ("RingText.Text"=w383:string)  [unwired: 2 in, 2 out]
    n217 = property on="内风机状态" class="Enum (strict)"() -> ("RingText.Text"=w382:string)  [unwired: 2 in, 2 out]
    n218 = property on="外风机状态" class="Enum (strict)"() -> ("RingText.Text"=w381:string)  [unwired: 2 in, 2 out]
    n219 = property on="加热状态" class="Enum (strict)"() -> ("RingText.Text"=w380:string)  [unwired: 2 in, 2 out]
    n220 = Bundle By Name(cluster=w392, "data.air_conditioner.air_conditioner.cabinet_temperature"=w387, "data.air_conditioner.air_conditioner.air_supply_temperature"=w386, "data.air_conditioner.air_conditioner.voltage"=w385, "data.air_conditioner.air_conditioner.current"=w384, "data.air_conditioner.air_conditioner.compressor_status"=w383, "data.air_conditioner.air_conditioner.Internal_fan_status"=w382, "data.air_conditioner.air_conditioner.external_fan_status"=w381, "data.air_conditioner.air_conditioner.heating_state"=w380, "data.air_conditioner.air_conditioner.refrigeration_state"=w378, "data.air_conditioner.air_conditioner.high_temperature_alarm"=w377, "data.air_conditioner.air_conditioner.low_temperature_alarm"=w376, "data.air_conditioner.air_conditioner.heater_fault"=w375, "data.air_conditioner.air_conditioner.temperature_sensor_fault"=w374, "data.air_conditioner.air_conditioner.high_voltage_alarm"=w373, "data.air_conditioner.air_conditioner.low_voltage_alarm"=w372, "data.air_conditioner.air_conditioner.refrigeration_start_point"=w370, "data.air_conditioner.air_conditioner.refrigeration_sensitive_point"=w369, "data.air_conditioner.air_conditioner.heating_start_point"=w368, "data.air_conditioner.air_conditioner.heating_sensitive_point"=w367, "data.air_conditioner.air_conditioner.high_temperature_alarm_point"=w366, "data.air_conditioner.air_conditioner.low_temperature_alarm_point"=w365, "data.air_conditioner.启用"=TRUE) -> (w389:T19)
    n221 = global write "工况数据接口全局.vi" "data"(w389) -> ()
  }
